vi "Set Default.vi"(11 "Relation in":refnum<class "Relation.lvclass">) -> (3 "Relation out":refnum<class "Relation.lvclass">)   [LabVIEW 2020, in "Conditum.lvlib" / "Columns.lvlib" / "Relation.lvclass"]
uses:
  Relation.lvclass
  Type/Type.lvclass
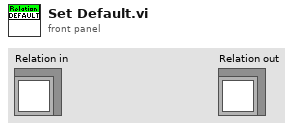
[diagram p1: front panel]
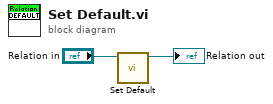
[diagram p0: block diagram]
diagram:
  n1 = call-parent "Set Default.vi"("Type in"="Relation in") -> ("Type out"=→"Relation out":refnum<class "Relation.lvclass">)  [unwired: 10 in]
